vi "Potting Data - BBM Pad Groups.vi"(8 "error in":errorcluster, 9 "Config Manager":refnum<class "Config Manager Class.lvclass">, 10 "Potting Selection BBM Bond Pads":bool[](array[boolean]), 11 "BBM Bond Pad References":T2[](array[typedef])) -> (0 "error out":errorcluster, 3 "Potting Lines":T1[](array[typedef]))   [LabVIEW 2011]
uses:
  Shared Components/Utils/Type Definitions/Fiducial Image.ctl
  Shared Components/Vec3d Class/Vec3d Class.lvclass
  Shared Components/Utils/Type Definitions/Physical Image.ctl
  <vilib>/vision/Image Controls.llb/IMAQ Image.ctl
  Shared Components/Utils/Type Definitions/Fiducial with Source.ctl
  Shared Components/Config Manager Class/Config Manager Class.lvclass
  Shared Components/Utils/Type Definitions/3d Line.ctl
  Shared Components/Config Manager Class/Type Definitions/Part Type.ctl
  Shared Components/Config Manager Class/Read Geometry Definition Integer.vi
  Shared Components/Config Manager Class/Read Geometry Definition Double.vi
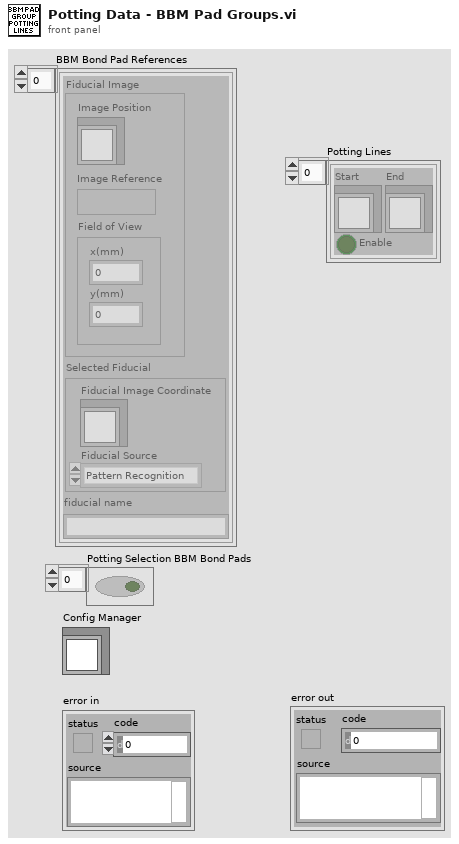
[diagram p1: front panel]
types:
  T1 = typedef "3d Line.ctl" = cluster{"Start":refnum<class "Vec3d Class.lvclass">, "End":refnum<class "Vec3d Class.lvclass">, "Enable":bool}
  T2 = typedef "Fiducial Image.ctl" = cluster{"Fiducial Image":T3, "Selected Fiducial":T5, "fiducial name":string}
  T3 = typedef "Physical Image.ctl" = cluster{"Image Position":refnum<class "Vec3d Class.lvclass">, "Image Reference":T4, "Field of View":cluster{"x(mm)":dbl, "y(mm)":dbl}}
  T4 = typedef "IMAQ Image.ctl" = refnum<image>
  T5 = typedef "Fiducial with Source.ctl" = cluster{"Fiducial Image Coordinate":refnum<class "Vec3d Class.lvclass">, "Fiducial Source":enum16{"Pattern Recognition", "User", "Error", "Default"}}
  T6 = typedef "Part Type.ctl" = enum16{"BBM", "HDI", "BARE HDI", "GLUERESERVOIR", "STAMP_1", "STAMP_2", "STAMP_3", "STAMP_4", "STAMP_5", "WEIGHT_1", "WEIGHT_2", "WEIGHT_3", "WEIGHT_4", "WEIGHT_5", "WEIGHT_6", "WEIGHT_7", "WEIGHT_8", "PICKER_TOOL", "GRABER_TOOL"}
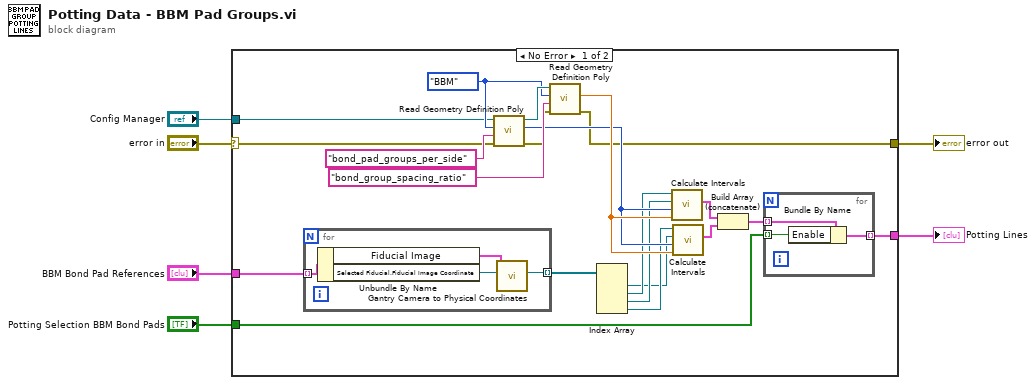
[diagram p0: block diagram]
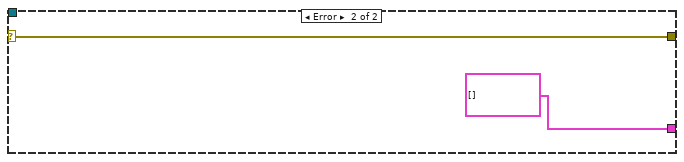
[diagram p2: hidden frame]
diagram:
  n1 = case shown="No Error" "error in" {
    selector: "error in" -> [w14 w36]
    tunnel: "Config Manager" -> [w23 _]
    tunnel: "BBM Bond Pad References" -> [w22 _]
    tunnel: "Potting Selection BBM Bond Pads" -> [w16 _]
    tunnel: [w7 T1[] [] ("appended array")] -> w2
    tunnel: [w12 w36] -> w1
    frame No Error {
      w26 = Part_Type."BBM" ("Part Type")
      n2 = for {
        tunnel: w22 -> [w34] mode=indexing
        tunnel: [w31] -> w21 mode=indexing
        n3 = Unbundle By Name(w34) -> ("Fiducial Image"=w33:T3, "Selected Fiducial.Fiducial Image Coordinate"=w32:refnum<class "Vec3d Class.lvclass">)
        n4 = call "Gantry Camera to Physical Coordinates.vi"("Image Coordinate"=w32, "Physical Image"=w33) -> ("Global Coordinate"=w31:refnum<class "Vec3d Class.lvclass">)  [unwired: 7 in, 2 out]
      }
      n5 = call-poly "Read Geometry Definition Poly.vi"("error in"=w14, "Feature"="bond_pad_groups_per_side", "Part Type"=w26, "Config Manager in"=w23) -> ("error out"=w13:errorcluster, "Geometry Definition"=w15:i32, "Config Manager out"=w27:refnum<class "Config Manager Class.lvclass">)  [unwired: 5 in]
      n6 = call-poly "Read Geometry Definition Poly.vi"("error in"=w13, "Feature"="bond_group_spacing_ratio", "Part Type"=w26, "Config Manager in"=w27) -> ("error out"=w12:errorcluster, "Geometry Definition"=w20:dbl)  [unwired: 5 in, 1 out]
      n7 = Index Array(array=w21) -> (element #1=w8:refnum<class "Vec3d Class.lvclass">, element #2=w10:refnum<class "Vec3d Class.lvclass">, element #3=w11:refnum<class "Vec3d Class.lvclass">, element #4=w9:refnum<class "Vec3d Class.lvclass">)  [unwired: 4 in]
      n8 = call "Calculate Intervals.vi"("gap/group ratio"=w20, "Num Intervals"=w15, "End"=w11, "Start"=w10) -> ("Intervals"=w19:T1[])  [unwired: 7 in]
      n9 = call "Calculate Intervals.vi"("gap/group ratio"=w20, "Num Intervals"=w15, "End"=w8, "Start"=w9) -> ("Intervals"=w18:T1[])  [unwired: 7 in]
      n10 = Build Array (concatenate)(w19, w18) -> (w17:T1[])
      n11 = for {
        tunnel: w17 -> [w30] mode=indexing
        tunnel: w16 -> [w29] mode=indexing
        tunnel: [w28] -> w7 mode=indexing
        n12 = Bundle By Name(cluster=w30, "Enable"=w29) -> (w28:T1)
      }
    }
    frame Error {
    }
  }
  "Potting Lines" <- w2
  "error out" <- w1
